vi "Close.vi"(0 "VISA resource name":refnum<visa-resource-name>, 11 "error in (no error)":errorcluster) -> (15 "error out":errorcluster)   [LabVIEW 2013, in "Stanford Research PS300 Series.lvlib"]
doc: "This VI closes the I/O interface with the instrument."
uses:
  Stanford Research PS300 Series.lvlib
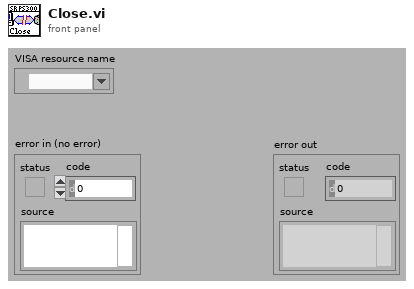
[diagram p1: front panel]
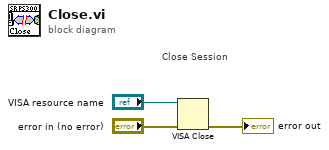
[diagram p0: block diagram]
diagram:
  # "Close Session"
  n1 = VISA Close(VISA resource name="VISA resource name", error in (no error)="error in (no error)") -> (error out=→"error out":errorcluster)
